vi "LocalizeKeyLowLevel.vi"(7 "Dictionary":T1, 8 "error in (no error)":errorcluster, 10 "Target Language":string, 11 "Key":string) -> (0 "error out":errorcluster, 3 "Localized Phrase":string)   [LabVIEW 2017, in "JKI Simple Localization.lvlib"]
uses:
  API/JKI Simple Localization.lvlib
  Definitions/Dictionary--Cluster.ctl
  Definitions/Private/FontCluster.ctl
  Definitions/Private/Phrase Dictionary.ctl
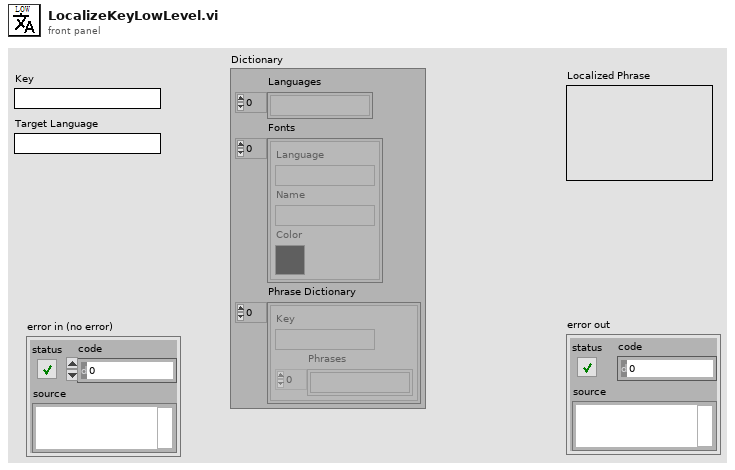
[diagram p1: front panel]
types:
  T1 = typedef "JKI Simple Localization.lvlib/Dictionary--Cluster.ctl" = cluster{"Languages":string[], "Fonts":T2[], "Phrase Dictionary":T3[]}
  T2 = typedef "JKI Simple Localization.lvlib/FontCluster.ctl" = cluster{"Language":string, "Name":string, "Color":u32}
  T3 = typedef "JKI Simple Localization.lvlib/Phrase Dictionary.ctl" = cluster{"Key":string, "Phrases":string[]}
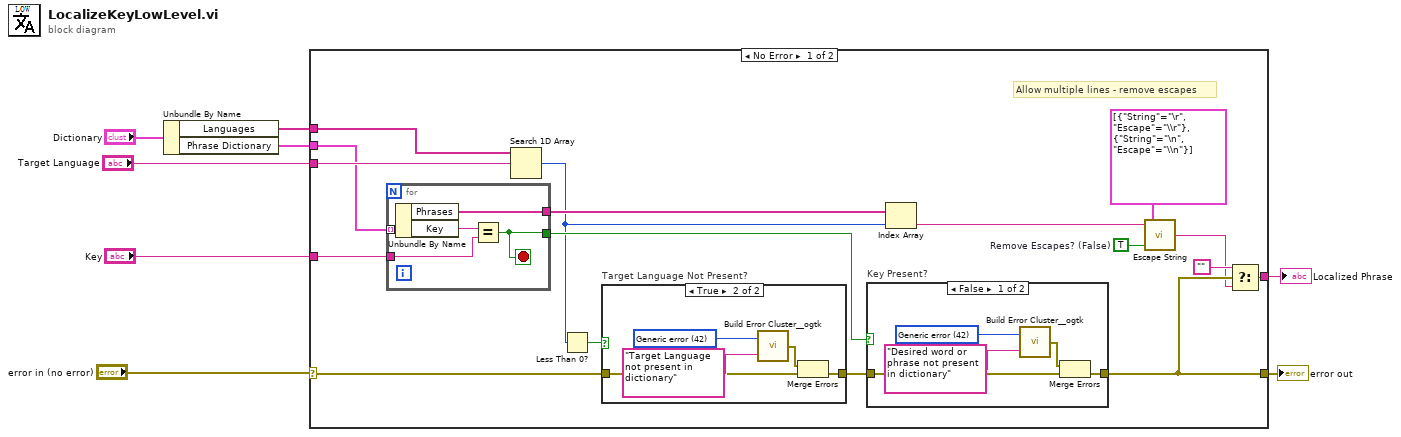
[diagram p0: block diagram]
diagram:
  n1 = Unbundle By Name("Dictionary") -> ("Languages"=w3:string[], "Phrase Dictionary"=w1:T3[])
  n2 = case shown="No Error" "error in (no error)" {
    selector: "error in (no error)" -> [w20 w43]
    tunnel: w3 -> [w25 _]
    tunnel: [w9 _] -> w8
    tunnel: [w12 w43] -> w7
    tunnel: "Target Language" -> [w19 _]
    tunnel: "Key" -> [w18 _]
    tunnel: w1 -> [w13 _]
    frame No Error {
      w22 = TRUE  # Remove Escapes? (False)
      # "Allow multiple lines - remove escapes"
      n3 = for {
        tunnel: w13 -> [w30] mode=indexing
        tunnel: w18 -> [w28]
        tunnel: [w27] -> w16
        tunnel: [w26] -> w17
        stop <- w27 stop-if-true
        n4 = Unbundle By Name(w30) -> ("Phrases"=w26:string[], "Key"=w29:string)
        n5 = Equal?(x=w29, y=w28) -> (x = y?=w27:bool)
      }
      n6 = Search 1D Array(1D array=w25, element=w19) -> (index of element=w15:i32)  [unwired: 1 in]
      n7 = Less Than 0?(x=w15) -> (x < 0?=w24:bool)
      n8 = case "Target Language Not Present?" shown="True" w24 {
        tunnel: w20 -> [w37 w39]
        tunnel: [w37 w38] -> w23
        frame False {
        }
        frame True {
          w42 = 42 items=["No error", "Argument error", "Memory is full", "Out of zone", "End of file", "File already open", "Generic file I/O error", "File not found", "File permission error", "Disk is full", "Duplicate path", "Too many files open", "System feature not enabled", "Resource file not found", "Cannot add resource", "Resource not found", "Image not found", "Image memory error", "Pen does not exist", "Config type invalid", "Config token not found", "Config parse error", "Config memory error", "Bad external code format", "Bad external code offset", "External code not present", "Null window", "Destroy window error", "Null menu", "Print aborted", "Bad print record", "Print driver error", "Windows error during printing", "Memory error during printing", "Print dialog error", "Generic print error", "Invalid device refnum", "Device not found", "Device parameter error", "Device unit error", "Cannot open device", "Device call aborted", "Generic error", "Cancelled by user", "Object ID too low", "Object ID too high", "Object not in heap", "Unknown heap", "Unknown object (invalid DefProc)", "Unknown object (DefProc not in table)", "Message out of range", "Invalid (null) method", "Unknown message", "Manager call not supported", "Bad address", "Network operation in progress", "Network operation timed out", "Connection is busy", "Network attribute not supported", "Network error", "Address in use", "System out of memory", "Connection aborted", "Connection refused", "Not connected", "Already connected", "Connection closed", "Initialization error (interapplication manager)", "Bad occurrence", "Wait on unbound occurrence handler", "Occurrence queue overflow", "Datalog type conflict", "Unused", "Unrecognized type (interapplication manager)", "Memory corrupt", "Failed to make temporary DLL", "Old CIN version", "Drag socket not found", "Failed to load drop-object", "Failed to register OLE object", "Failed to release OLE object", "Format specifier type mismatch", "Unknown format specifier", "Too few format specifiers", "Too many format specifiers", "Scan failed", "Newer CIN version", "Error converting to variant", "Runtime menu error", "Password tampered", "Variant attribute not found", "Incompatible variant data type", "Event data is not available", "Event Store is not present", "Occurrence is not found", "Event Queue is not created", "Event info is not available", "Refnum passed is NULL", "Error retrieving Class GUID", "Error retrieving CoClass GUID", "Error retrieving TypeLib GUID.", "Bad built application magic bytes.", "Specific driver is different from the specific driver associated with the Logical Name.", "There is no session opened to the class driver.", "Max Error", "MAX - Error with config objects", "MAX - Error loading configuration", "MAX - Group not supported"]
          n9 = call <userlib>:"Build Error Cluster__ogtk.vi"("String to Prepend to source (\"\")"="Target Language not present in dictionary" ("String to Prepend to source (\"\")"), "code"=w42) -> ("error out"=w40:errorcluster)
          n10 = Merge Errors(w40, w39) -> (w38:errorcluster)
        }
      }
      n11 = case "Key Present?" shown="False" w16 {
        tunnel: w23 -> [w32 w36]
        tunnel: [w31 w36] -> w12
        frame False {
          w35 = 42 items=["No error", "Argument error", "Memory is full", "Out of zone", "End of file", "File already open", "Generic file I/O error", "File not found", "File permission error", "Disk is full", "Duplicate path", "Too many files open", "System feature not enabled", "Resource file not found", "Cannot add resource", "Resource not found", "Image not found", "Image memory error", "Pen does not exist", "Config type invalid", "Config token not found", "Config parse error", "Config memory error", "Bad external code format", "Bad external code offset", "External code not present", "Null window", "Destroy window error", "Null menu", "Print aborted", "Bad print record", "Print driver error", "Windows error during printing", "Memory error during printing", "Print dialog error", "Generic print error", "Invalid device refnum", "Device not found", "Device parameter error", "Device unit error", "Cannot open device", "Device call aborted", "Generic error", "Cancelled by user", "Object ID too low", "Object ID too high", "Object not in heap", "Unknown heap", "Unknown object (invalid DefProc)", "Unknown object (DefProc not in table)", "Message out of range", "Invalid (null) method", "Unknown message", "Manager call not supported", "Bad address", "Network operation in progress", "Network operation timed out", "Connection is busy", "Network attribute not supported", "Network error", "Address in use", "System out of memory", "Connection aborted", "Connection refused", "Not connected", "Already connected", "Connection closed", "Initialization error (interapplication manager)", "Bad occurrence", "Wait on unbound occurrence handler", "Occurrence queue overflow", "Datalog type conflict", "Unused", "Unrecognized type (interapplication manager)", "Memory corrupt", "Failed to make temporary DLL", "Old CIN version", "Drag socket not found", "Failed to load drop-object", "Failed to register OLE object", "Failed to release OLE object", "Format specifier type mismatch", "Unknown format specifier", "Too few format specifiers", "Too many format specifiers", "Scan failed", "Newer CIN version", "Error converting to variant", "Runtime menu error", "Password tampered", "Variant attribute not found", "Incompatible variant data type", "Event data is not available", "Event Store is not present", "Occurrence is not found", "Event Queue is not created", "Event info is not available", "Refnum passed is NULL", "Error retrieving Class GUID", "Error retrieving CoClass GUID", "Error retrieving TypeLib GUID.", "Bad built application magic bytes.", "Specific driver is different from the specific driver associated with the Logical Name.", "There is no session opened to the class driver.", "Max Error", "MAX - Error with config objects", "MAX - Error loading configuration", "MAX - Group not supported"]
          n12 = call <userlib>:"Build Error Cluster__ogtk.vi"("String to Prepend to source (\"\")"="Desired word or phrase not present in dictionary" ("String to Prepend to source (\"\")"), "code"=w35) -> ("error out"=w33:errorcluster)
          n13 = Merge Errors(w33, w32) -> (w31:errorcluster)
        }
        frame True {
        }
      }
      n14 = Index Array(array=w17, index=w15) -> (element=w14:string)
      n15 = call <vilib>:"Escape String.vi"("Remove Escapes? (False)"=w22, "Escapes"=cluster{"String":string, "Escape":string}[] [{"String"="\r", "Escape"="\\r"}, {"String"="\n", "Escape"="\\n"}], "String in"=w14) -> ("String out"=w10:string)
      n16 = Select(t="", s=w12, f=w10) -> (s? t:f=w9:string)
    }
    frame Error {
    }
  }
  "Localized Phrase" <- w8
  "error out" <- w7
